vi "Reset Status.vi"(10 "Run Queue":set{string}(c389), 11 "Result Model In":refnum<class "Result Model.lvclass">) -> (3 "Result Model Out":refnum<class "Result Model.lvclass">)   [LabVIEW 2020, in "Result Model.lvclass"]
uses:
  Result Model.lvclass
  Result Model.lvclass/Result Model.ctl
  Core/Result/Status.ctl
  Core/Result/Result.lvlib
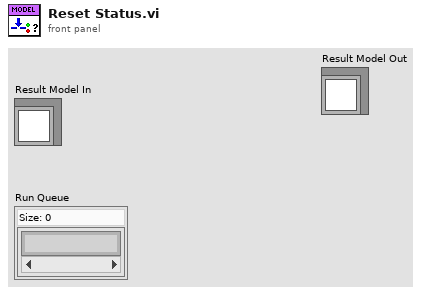
[diagram p1: front panel]
types:
  T1 = typedef "Result.lvlib/Status.ctl" = enum16{"", "Passed", "Failed", "Error", "Skipped", "Setup Error", "Broken", "Teardown Error"}
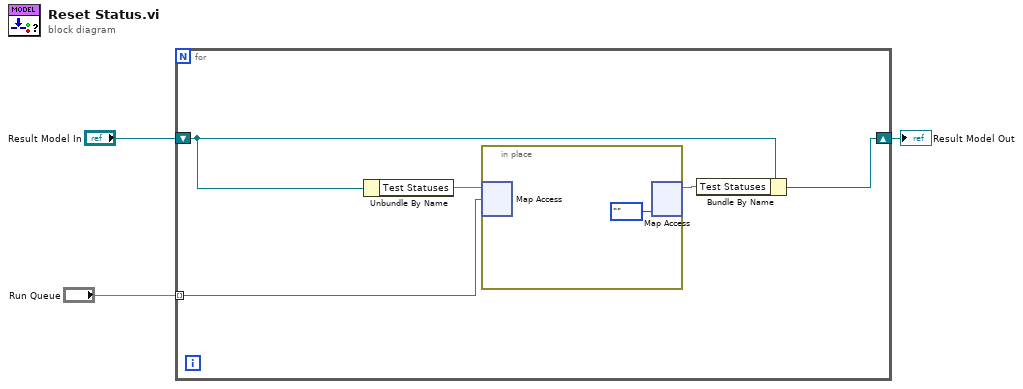
[diagram p0: block diagram]
diagram:
  n1 = for {
    tunnel: "Run Queue" -> [w8] mode=indexing
    shift-right: [w4] -> w1
    shift-left: "Result Model In" -> [w5]
    n2 = Unbundle By Name(w5) -> ("Test Statuses"=w7:map{string, T1})
    n3 = in-place {
      n4 = in-place-map #1(w7, w8) -> ()  [unwired: 1 in, 2 out]
      n5 = in-place-map #1(Status."" ("value")) -> (w6:map{string, T1})  [unwired: 1 in, 2 out]
    }
    n6 = Bundle By Name(cluster=w5, "Test Statuses"=w6) -> (w4:refnum<class "Result Model.lvclass">)
  }
  "Result Model Out" <- w1
